vi "Demo_obtain_value_selected.vi"(10 "index (row)":i32, 11 "MulticolumnListbox in":refnum<vi>) -> (2 "element":string)   [LabVIEW 2019, in "Nestle_Actor.lvlib" / "Nestle_Actor.lvclass"]
uses:
  Nestle_Actor.lvclass
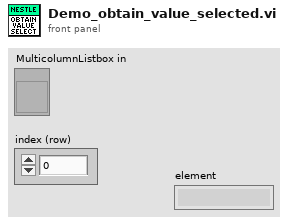
[diagram p1: front panel]
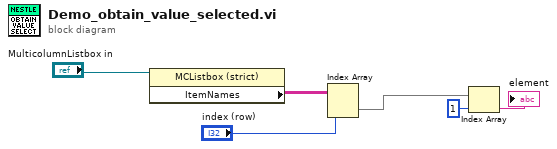
[diagram p0: block diagram]
diagram:
  n1 = property class="MCListbox (strict)"(reference="MulticolumnListbox in") -> ("ItemNames"=w5:string[][])  [unwired: 1 in, 2 out]
  n2 = Index Array(array=w5, index (row)="index (row)") -> (element=w2:string[])  [unwired: 1 in]
  n3 = Index Array(array=w2, index=1) -> (element=→"element":string)
